vi "TB-Analyze.vi"(1 "state in":T1, 9 "AI Waveforms":dbl[][](array[numeric]), 11 "error in (no error)":errorcluster, 12 "Exposure parameters":T4={"Low cutoff (kHz)"=0.0, "High cutoff (kHz)"=0.0, "Duration (min)"=0.0, "dB SPL"=100.0, "Waveform"=enum."Noise", "WAVfile"=path "", "refWav"=path "", "use mic correction"=FALSE, "micCorrFile"=path "", "Pistonphone Level (dB SPL)"=0.0, "Sampling rate (Hz)"=0.0, "Buffer length (s)"=0.0, "Stream mic"=FALSE, "Fine adjust"={"Max"=0.0, "Min"=0.0}, "Mic gain"=0.0, "atten"=0.0, "resol (Hz)"=0.0, "navgs"=0, "Allow Slack"=FALSE, "max starts"=0, "Freq (kHz)"=8.0, "Tma (s)"=0.0, "Streamed"=[], "Drive"=""}, 13 "Pistonphone Factor":dbl) -> (3 "state out":T1, 4 "waveform":waveform(dbl), 6 "spectrum":waveform(dbl), 8 "Overload":bool, 10 "Cal SPL":dbl, 14 "history values":dbl[](array[numeric]), 15 "error out":errorcluster)   [LabVIEW 2020]
uses:
  Typedefs/TB-Parameters.ctl
  epl-vi-lib/Signal Synthesis VIs/Controls/Waveform XCtl/Waveform Enum.ctl
  Typedefs/TB-Runtime state.ctl
  <vilib>/sound2/lvsound2.llb/Sound File Refnum.ctl
  Typedefs/TB-Setup Log.ctl
  <vilib>/Analysis/5stat.llb/RMS (DBL).vi
  <vilib>/Analysis/baseanly.llb/Mean.vi
  <vilib>/Analysis/baseanly.llb/Mean (DBL).vi
  epl-vi-lib/Utility VIs/Math VIs/Linear to dB (scalar).vi
  epl-vi-lib/Utility VIs/Math VIs/FFT x(t) to dB,Degrees (1D).vi
  epl-vi-lib/Utility VIs/Math VIs/dB to Linear (1D).vi
  <vilib>/Analysis/NI_AALPro.lvlib
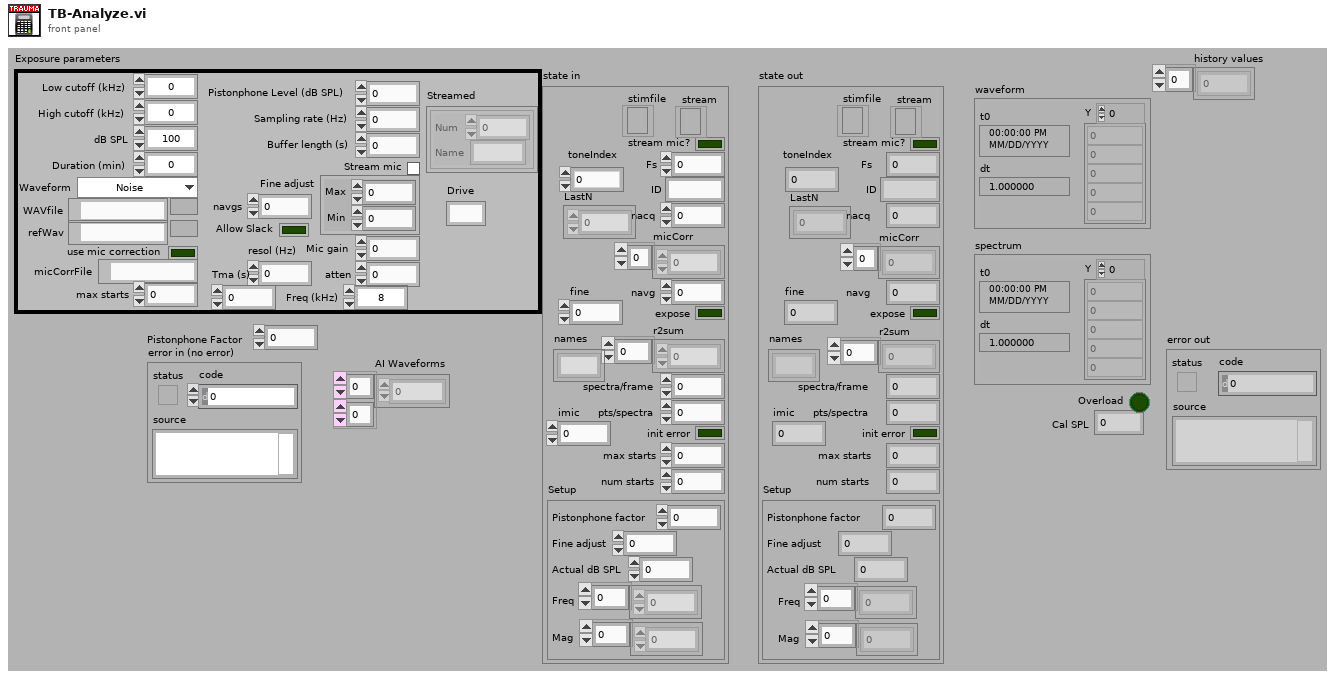
[diagram p1: front panel]
types:
  T1 = typedef "TB-Runtime state.ctl" = cluster{"stimfile":T2, "stream mic?":bool, "Fs":dbl, "ID":string, "micCorr":dbl[], "navg":i32, "r2sum":dbl[], "expose":bool, "spectra/frame":i32, "pts/spectra":i32, "nacq":i32, "init error":bool, "max starts":i32, "num starts":i32, "Setup":T3, "toneIndex":i32, "LastN":dbl[], "fine":dbl, "imic":i32, "stream":refnum<file>, "names":string[]}
  T2 = typedef "Sound File Refnum.ctl" = refnum<file>
  T3 = typedef "TB-Setup Log.ctl" = cluster{"Pistonphone factor":dbl, "Fine adjust":dbl, "Actual dB SPL":dbl, "Freq":dbl[], "Mag":dbl[]}
  T4 = typedef "TB-Parameters.ctl" = cluster{"Low cutoff (kHz)":dbl, "High cutoff (kHz)":dbl, "Duration (min)":dbl, "dB SPL":dbl, "Waveform":T5, "WAVfile":path, "refWav":path, "use mic correction":bool, "micCorrFile":path, "Pistonphone Level (dB SPL)":dbl, "Sampling rate (Hz)":dbl, "Buffer length (s)":dbl, "Stream mic":bool, "Fine adjust":cluster{"Max":dbl, "Min":dbl}, "Mic gain":dbl, "atten":dbl, "resol (Hz)":dbl, "navgs":i32, "Allow Slack":bool, "max starts":i32, "Freq (kHz)":dbl, "Tma (s)":dbl, "Streamed":cluster{"Num":i32, "Name":string}[], "Drive":string}
  T5 = typedef "Waveform Enum.ctl" = enum16{"OFF", "Tone", "Noise", "Pulse Train", "File", "FM Sweep", "Chirp Train", "Complex Tone", "FM Tone", "Moving Ripple"}
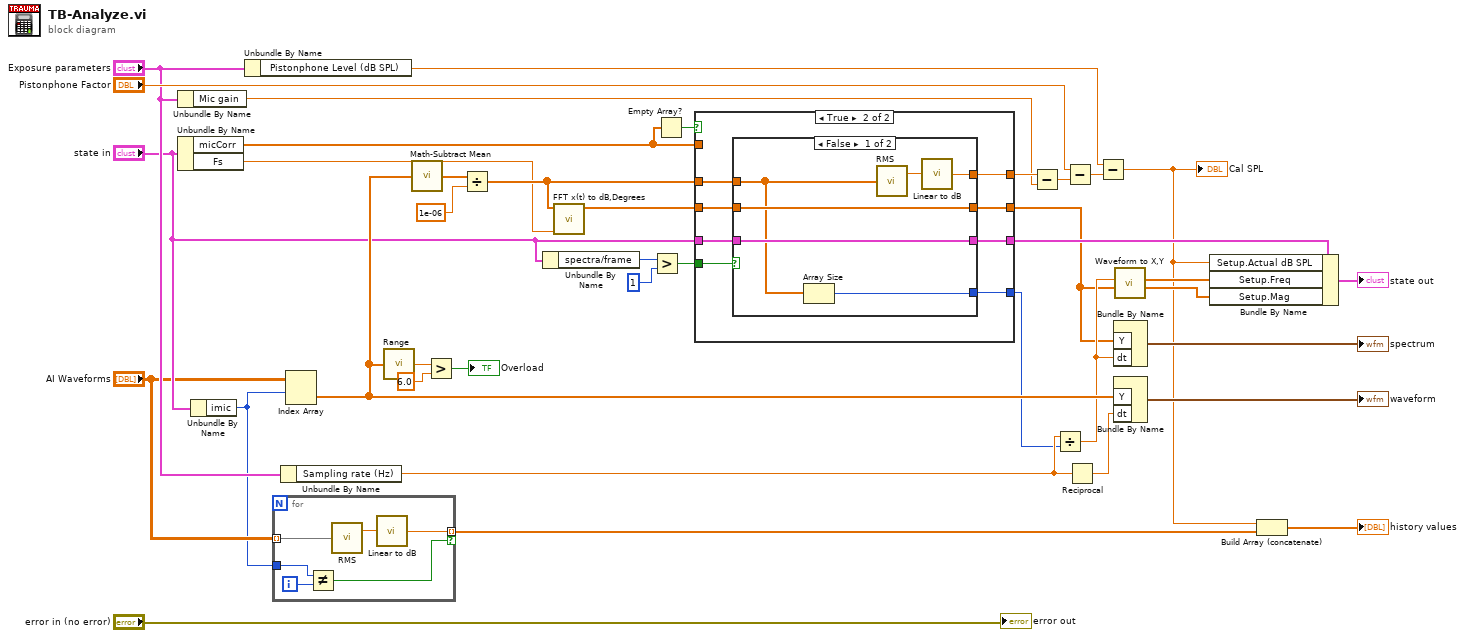
[diagram p0: block diagram]
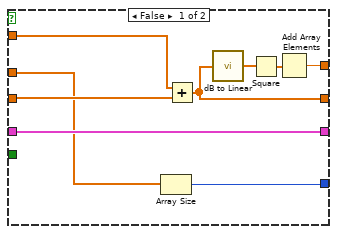
[diagram p2: hidden frame]
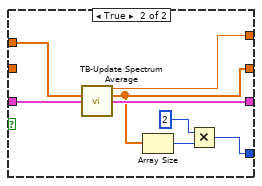
[diagram p3: hidden frame]
diagram:
  n1 = Unbundle By Name("Exposure parameters") -> ("Mic gain"=w21:dbl)
  n2 = Unbundle By Name("state in") -> ("micCorr"=w13:dbl[], "Fs"=w22:dbl)
  n3 = Unbundle By Name("state in") -> ("imic"=w4:i32)
  n4 = Unbundle By Name("Exposure parameters") -> ("Pistonphone Level (dB SPL)"=w31:dbl)
  n5 = for {
    tunnel: "AI Waveforms" -> [w44] mode=indexing
    tunnel: [w43] -> w3 mode=indexing if=w40
    tunnel: w4 -> [w41]
    i -> [w42]
    n6 = Not Equal?(x=w41, y=w42) -> (x != y?=w40:bool)
    n7 = call-poly <vilib>:"RMS.vi"("X"=w44) -> ("rms value"=w45:dbl)  [unwired: 1 out]
    n8 = call-poly "Linear to dB.vi"("Linear"=w45) -> ("dB"=w43:dbl)
  }
  n9 = Unbundle By Name("Exposure parameters") -> ("Sampling rate (Hz)"=w30:dbl)
  n10 = Index Array(array="AI Waveforms", index (row)=w4) -> (element=w35:dbl[])  [unwired: 1 in]
  n11 = call "Range.vi"("Array"=w35) -> ("Range"=w34:dbl)
  n12 = call "Math-Subtract Mean.vi"("Y"=w35) -> ("Y - mean(Y)"=w15:dbl[])  [unwired: 4 in]
  n13 = Greater?(x=w34, y=6.0) -> (0:→"Overload":bool)
  n14 = Divide(x=w15, y=1e-06) -> (x/y=w25:dbl[])
  n15 = Unbundle By Name("state in") -> ("spectra/frame"=w19:i32)
  n16 = call-poly "FFT x(t) to dB,Degrees.vi"("Fs (Hz)"=w22, "X"=w25) -> ("+Freq. Mag of FFT (dB rms)"=w24:dbl[])  [unwired: 7 in, 2 out]
  n17 = Greater?(x=w19, y=1) -> (0:w18:bool)
  n18 = Empty Array?(array=w13) -> (empty?=w14:bool)
  n19 = case shown="True" w14 {
    tunnel: [w50 w62] -> w26
    tunnel: w25 -> [w47 w61]
    tunnel: w13 -> [w49 _]
    tunnel: w24 -> [w54 w59]
    tunnel: [w53 w60] -> w7
    tunnel: "state in" -> [w48 w58]
    tunnel: [w48 w57] -> w23
    tunnel: w18 -> [_ w56]
    tunnel: [w46 w55] -> w16
    frame False {
      n20 = Array Size(array=w47) -> (size(s)=w46:i32)
      n21 = Add(x=w49, y=w54) -> (x+y=w53:dbl[])
      n22 = call-poly "dB to Linear.vi"("dB"=w53) -> ("linear"=w51:dbl[])
      n23 = Square(x=w51) -> (x^2=w52:dbl[])
      n24 = Add Array Elements(numeric array=w52) -> (sum=w50:dbl)
    }
    frame True {
      n25 = case shown="False" w56 {
        tunnel: [w68 w76] -> w62
        tunnel: w61 -> [w64 w69]
        tunnel: [w66 w73] -> w60
        tunnel: w59 -> [w66 _]
        tunnel: w58 -> [w65 w74]
        tunnel: [w65 w75] -> w57
        tunnel: [w63 w70] -> w55
        frame False {
          n26 = Array Size(array=w64) -> (size(s)=w63:i32)
          n27 = call-poly <vilib>:"RMS.vi"("X"=w64) -> ("rms value"=w67:dbl)  [unwired: 1 out]
          n28 = call-poly "Linear to dB.vi"("Linear"=w67) -> ("dB"=w68:dbl)
        }
        frame True {
          n29 = call "TB-Update Spectrum Average.vi"("mic signal"=w69, "state in"=w74) -> ("RMS"=w76:dbl, "+Freq. Mag of FFT (dB rms) out"=w73:dbl[], "state out"=w75:T1)  [unwired: 11 in]
          n30 = Array Size(array=w73) -> (size(s)=w72:i32)
          n31 = Multiply(x=2, y=w72) -> (x*y=w70:i32)
        }
      }
    }
  }
  n32 = Subtract(x=w26, y=w21) -> (x-y=w28:dbl)
  n33 = Divide(x=w30, y=w16) -> (x/y=w8:dbl)
  n34 = Subtract(x="Pistonphone Factor", y=w28) -> (x-y=w29:dbl)
  n35 = Reciprocal(x=w30) -> (1/x=w38:dbl)
  n36 = Subtract(x=w31, y=w29) -> (x-y=w1:dbl)
  "Cal SPL" <- w1
  n37 = Bundle By Name("Y"=w7, "dt"=w8) -> (→"spectrum":waveform(dbl))  [unwired: 1 in]
  n38 = Bundle By Name("Y"=w35, "dt"=w38) -> (→"waveform":waveform(dbl))  [unwired: 1 in]
  n39 = call "Waveform to X,Y.vi"("Y"=w7, "dx"=w8) -> ("Y"=w9:dbl[], "X"=w10:dbl[])  [unwired: 5 in]
  n40 = Bundle By Name(cluster=w23, "Setup.Actual dB SPL"=w1, "Setup.Freq"=w10, "Setup.Mag"=w9) -> (→"state out":T1)
  n41 = Build Array (concatenate)(w1, w3) -> (→"history values":dbl[])
  "error out" <- "error in (no error)"
